vi "Drive Published Globals.vi"() -> ()   [LabVIEW 2015]
doc: "This is used primarily to publish values that other subsystems or user code may want to read periodically. It may also contain some settings such as debug switches or implementation selections that are independent of the operating mode of the subsystem."
uses:
  Support Code/Team900-VIs/navX Library v2/TypeDefs/Z900_navX_DeviceTypeDef.ctl
  Support Code/Team900-VIs/navX Library v2/TypeDefs/Z900_navX_ProtocolTypeDef.ctl
  Support Code/Team900-VIs/navX Library v2/TypeDefs/Z900_navX_NotifyPacketTypeDef.ctl
  Support Code/Team900-VIs/navX Library v2/TypeDefs/Z900_navX_ActionTypeDef.ctl
  Support Code/Team900-VIs/navX Library v2/navX Library v2.lvlib
panel:
  out "Operation Finished?":bool
  in  "navX Device":T1={"Interface"={"Protocol"=enum."SERIAL", "Update Rate (4Hz-60Hz)"=4, "navX Open TypeDef"=variant}, "Notify Packet"=refnum, "Loop VI Refnum"=refnum, "Ready to Close Occurrence Refnum"=refnum} {"Interface"."Update Rate (4Hz-60Hz)" min=4 max=60 step=1}
  in  "Drive Train Length (Front to Back)":dbl=31.0
  in  "Drive Train Width (wheel to wheel)":dbl=28.5
  in  "Encoder Right":dbl
  in  "Encoder Left":dbl
  # "Tip: The global is a good way publish state or\ninformational/debugging values.\nIt is not  advised that you put setpoint values here."
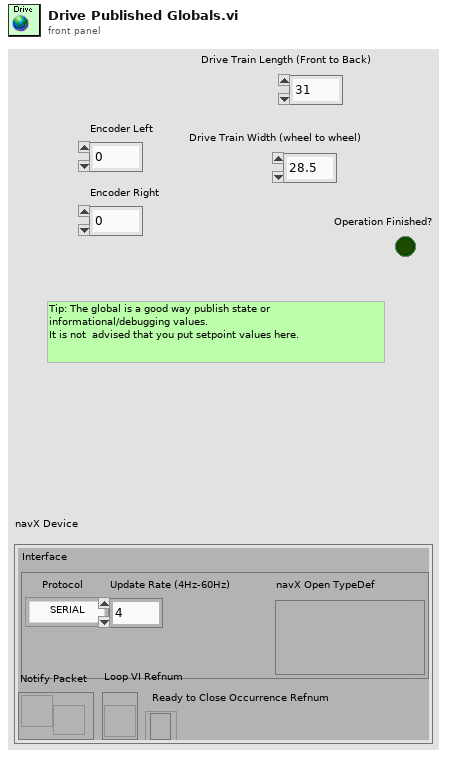
[diagram p1: front panel]
types:
  T1 = typedef "navX Library v2.lvlib/Z900_navX_DeviceTypeDef.ctl" = cluster{"Interface":cluster{"Protocol":T2, "Update Rate (4Hz-60Hz)":u8, "navX Open TypeDef":variant}, "Notify Packet":refnum<notifier>, "Loop VI Refnum":refnum<vi>, "Ready to Close Occurrence Refnum":refnum<k4>}
  T2 = typedef "navX Library v2.lvlib/Z900_navX_ProtocolTypeDef.ctl" = enum16{"SERIAL", "I2C", "SPI"}
diagram:
